vi "TIFF_XMP.vi"() -> ()   [LabVIEW 2025]
panel:
  in  "error in (no error)":errorcluster
  out "error out":errorcluster
  in  "XMP":string
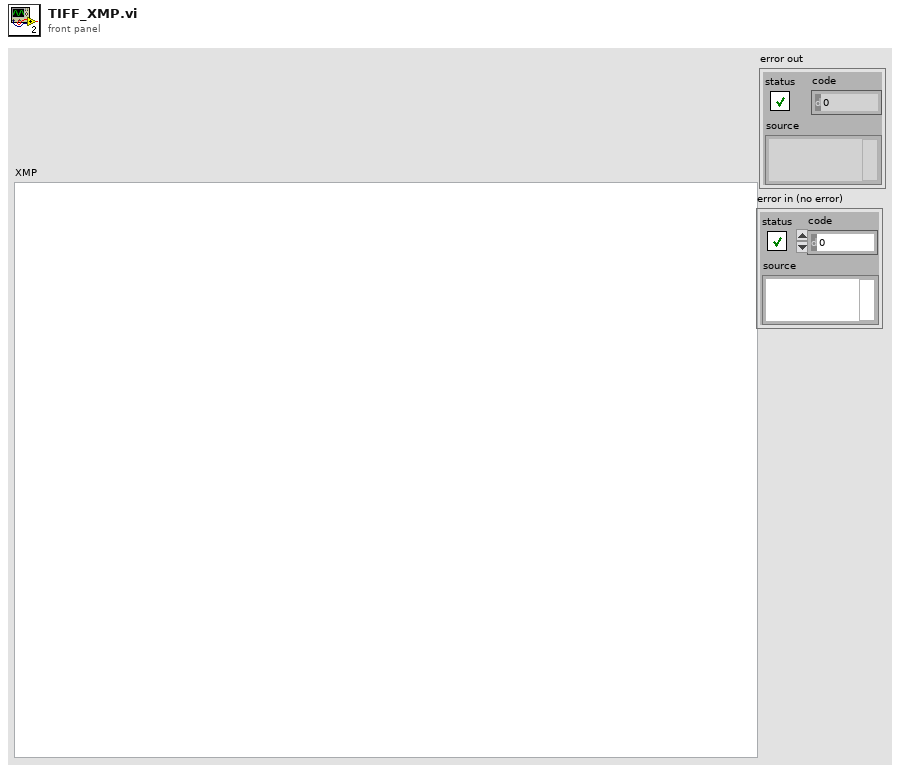
[diagram p1: front panel]
types:
  T1 = enum16{"open", "replace", "create", "open or create", "replace or create", "replace or create with confirmation"}
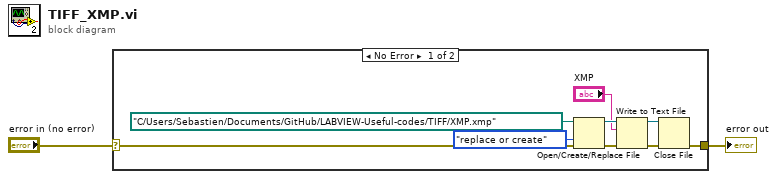
[diagram p0: block diagram]
diagram:
  n1 = case shown="No Error" "error in (no error)" {
    selector: "error in (no error)" -> [w10 w12]
    tunnel: [w4 w12] -> w2
    frame No Error {
      n2 = Open/Create/Replace File(file path (use dialog)=path "C:/Users/Sebastien/Documents/GitHub/LABVIEW-Useful-codes/TIFF/XMP.xmp", error in=w10, operation (0:open)=T1."replace or create") -> (refnum out=w9:refnum<file>, error out=w8:errorcluster)  [unwired: 3 in, 1 out]
      n3 = Write to Text File(file (use dialog)=w9, text="XMP", error in=w8) -> (refnum out=w6:refnum<file>, error out=w5:errorcluster)  [unwired: 1 in, 1 out]
      n4 = Close File(refnum=w6, error in=w5) -> (error out=w4:errorcluster)  [unwired: 1 out]
    }
    frame Error {
    }
  }
  "error out" <- w2
